vi "GetXMenuData.vi"(8 "error in (no error)":errorcluster, 11 "CMenu in":refnum<class "CMenu.lvclass">) -> (0 "error out":errorcluster, 2 "Items":T1(array[cluster]), 3 "CMenu out":refnum<class "CMenu.lvclass">)   [LabVIEW 2020, in "CMenu.lvclass"]
uses:
  CMenu.lvclass
  CMenu.lvclass/CMenu.ctl
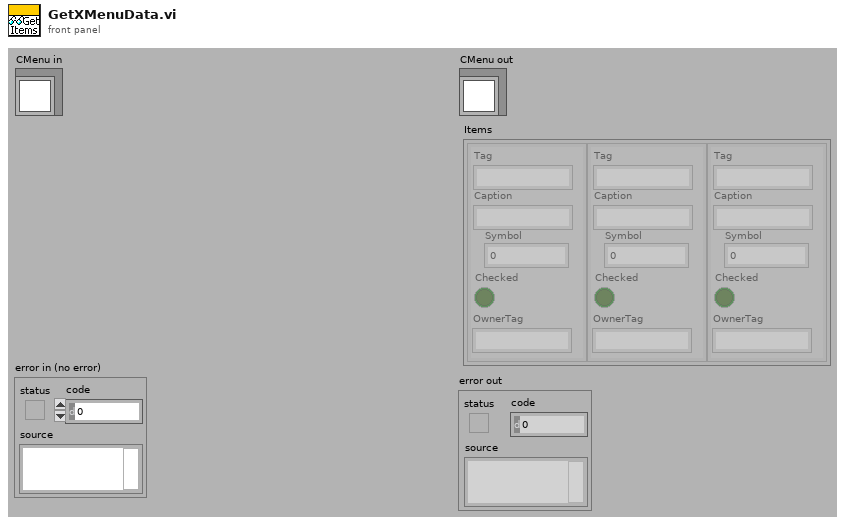
[diagram p1: front panel]
types:
  T1 = cluster{"Tag":string, "Caption":string, "Symbol":i32, "Checked":bool, "OwnerTag":string}[]
  T2 = cluster{"Tag":string, "Name":string, "Symbol":i32, "Checked":bool, "ParentTag":string}[]
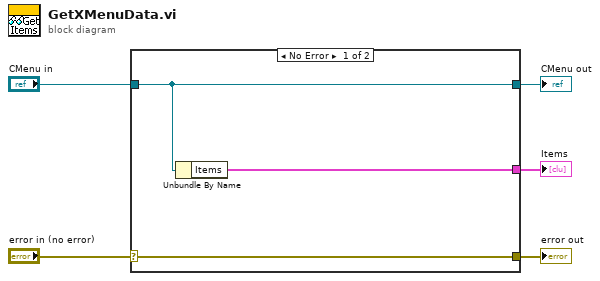
[diagram p0: block diagram]
diagram:
  n1 = case shown="No Error" "error in (no error)" {
    selector: "error in (no error)" -> [w8 w9]
    tunnel: [w8 w9] -> w4
    tunnel: [w7 w10] -> w2
    tunnel: "CMenu in" -> [w7 w10]
    tunnel: [w6 _] -> w1
    frame No Error {
      n2 = Unbundle By Name(w7) -> ("Items"=w6:T2)
    }
    frame Error {
    }
  }
  "error out" <- w4
  "CMenu out" <- w2
  "Items" <- w1
